vi "tensiletestpractice.vi"() -> ()   [LabVIEW 2014]
uses:
  <vilib>/Motion/FlexMotion/CustomControls/CustomControls.llb/Axis To Control.flx
  <vilib>/Motion/FlexMotion/FunctionsVIs/StartStopMotion.llb/Start Motion (8 axes).flx
  <vilib>/Motion/FlexMotion/FunctionsVIs/Trajectory.llb/Check Move Complete Status (8 axes).flx
  <vilib>/Motion/FlexMotion/FunctionsVIs/StartStopMotion.llb/Stop Motion (8 axes).flx
  Instance           1 22Saved   membrane_test3 .vi
  <vilib>/addons/_office/excel.llb/Excel Easy Table (num).vi
  <vilib>/Utility/NIReport.llb/NI_report.lvclass
  <vilib>/vision/NI_Vision_Development_Module.lvlib
  <vilib>/addons/_office/NI_ReportGenerationToolkit.lvlib
panel:
  out "?":string
  in  "Zero":dbl=-99.6 format="%#_13g"
  in  "Stretch Ratio Muliplier Per Cycle After":dbl=1.0 min=1.0
  in  "Number of cycles at 1x stretch ratio":dbl
  out "Waveform Chart":dynamicdata(graph)
  out "Finished at (s)":dbl format="%0.3f"
  in  "?":bool
  in  "Input File Path":path=path "C:/Users/aldasou3.ME204/Desktop/information.txt"
  out "Stretch length (mm)":dbl
  out "Estimated time from\nStart to finish (s)":dbl
  out "Elapsed Time (s)":dbl format="%0.3f"
  in  "Number of cycles":dbl
  in  "Stretch ratio":dbl
  in  "Motor speed\n(mm/s)":dbl
  in  "Undeformed\nLength (mm)\n(post to post)":dbl
  out "Voltage(V)":dbl=0.3869919147841388
  out "Particle Coordinates":dbl[][](array[numeric])
  out "Force (grams)":dbl=0.3869919147841388
  out "Selected Region of Interest":T1(plugin-control)
  out "Binary/ Segmented Image":T1(plugin-control)
  # "Michigan State University\nDepartment of Mechanical Engineering\nSoft Tissues Research Laboratory"
  # "Tensile Test and Particle Tracking VI"
  # "Image  Acquisition and Processing"
  # "Motion Control"
  # "Inputs"
  # "Selected Region of Interest"
  # "Experimental Data"
  # "Binary/Segmented Image"
  # "Distance between dots(mm)"
  # "1"
  # "2"
  # "3"
  # "4"
  # "Button must be white to run"
  # "5"
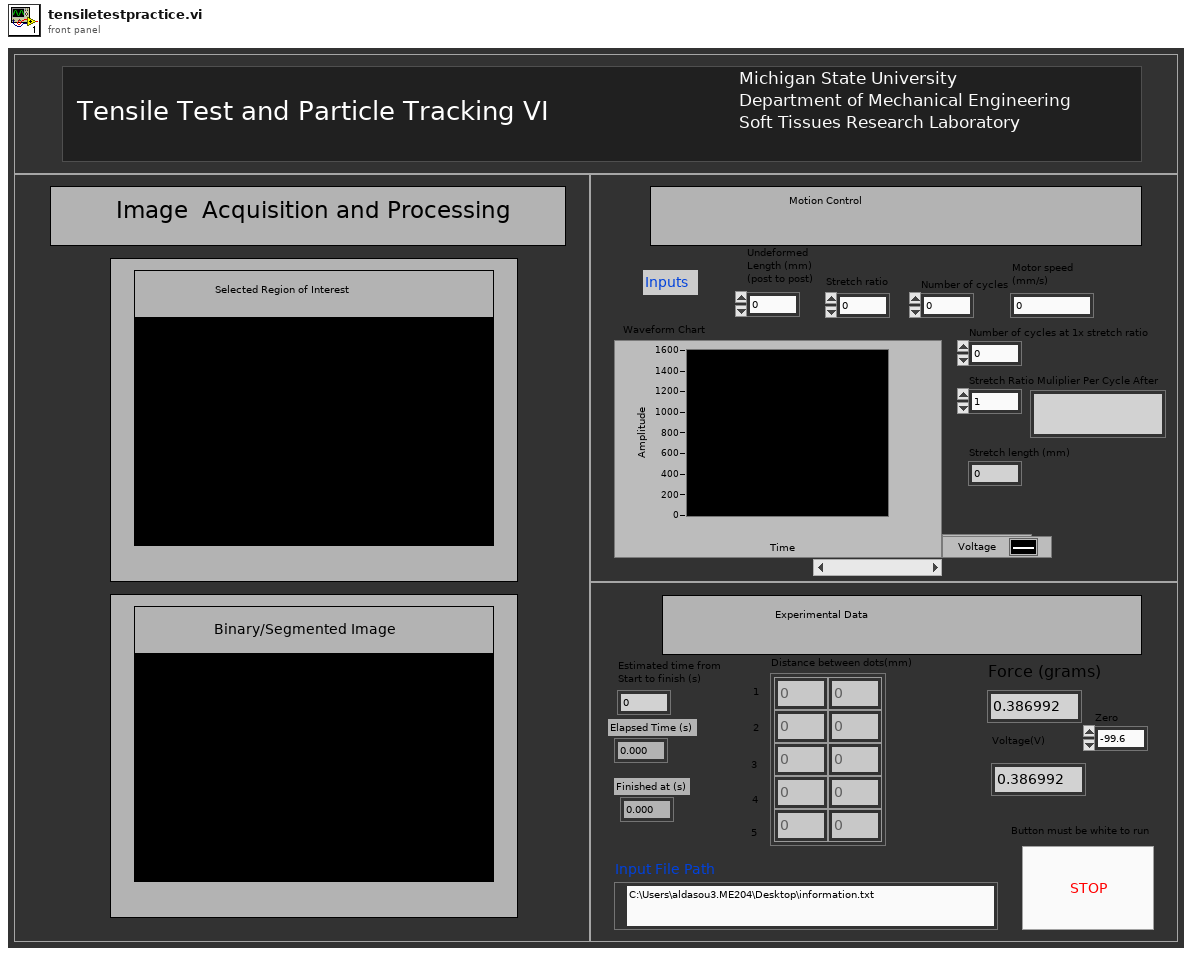
[diagram p1: front panel]
types:
  T1 = typedef "IMAQ Image.ctl" = refnum<image>
  T2 = typedef "Board Id" = u8
  T3 = enum16{"Absolute Position", "Relative Position", "Velocity", "Relative to Cap Pos", "Modulus Position", "Absolute Contouring", "Relative Contouring"}
  T4 = enum16{"Standard Report", "HTML", "Word", "Excel"}
  T5 = typedef "ROI Descriptor" = cluster{"Global Rectangle":i32[], "Contours":cluster{"ID":enum32{"External", "Internal"}, "Type":u32, "Coordinates":i32[]}[]}
  T6 = typedef "Axis To Control.flx" = u16
  T7 = typedef "Bd Id Out" = u8
  T8 = typedef "Resource Out (Enum).flx" = u16
  T9 = typedef "LVDateTimeRec.ctl" = cluster{"fractional second":dbl, "second":i32, "minute":i32, "hour":i32, "day of month":i32, "month":i32, "year":i32, "day of week":i32, "day of year":i32, "DST":i32}
  T10 = cluster{"month":i32, "day of month":i32, "year":i32, "hour":i32, "minute":i32, "second":i32}
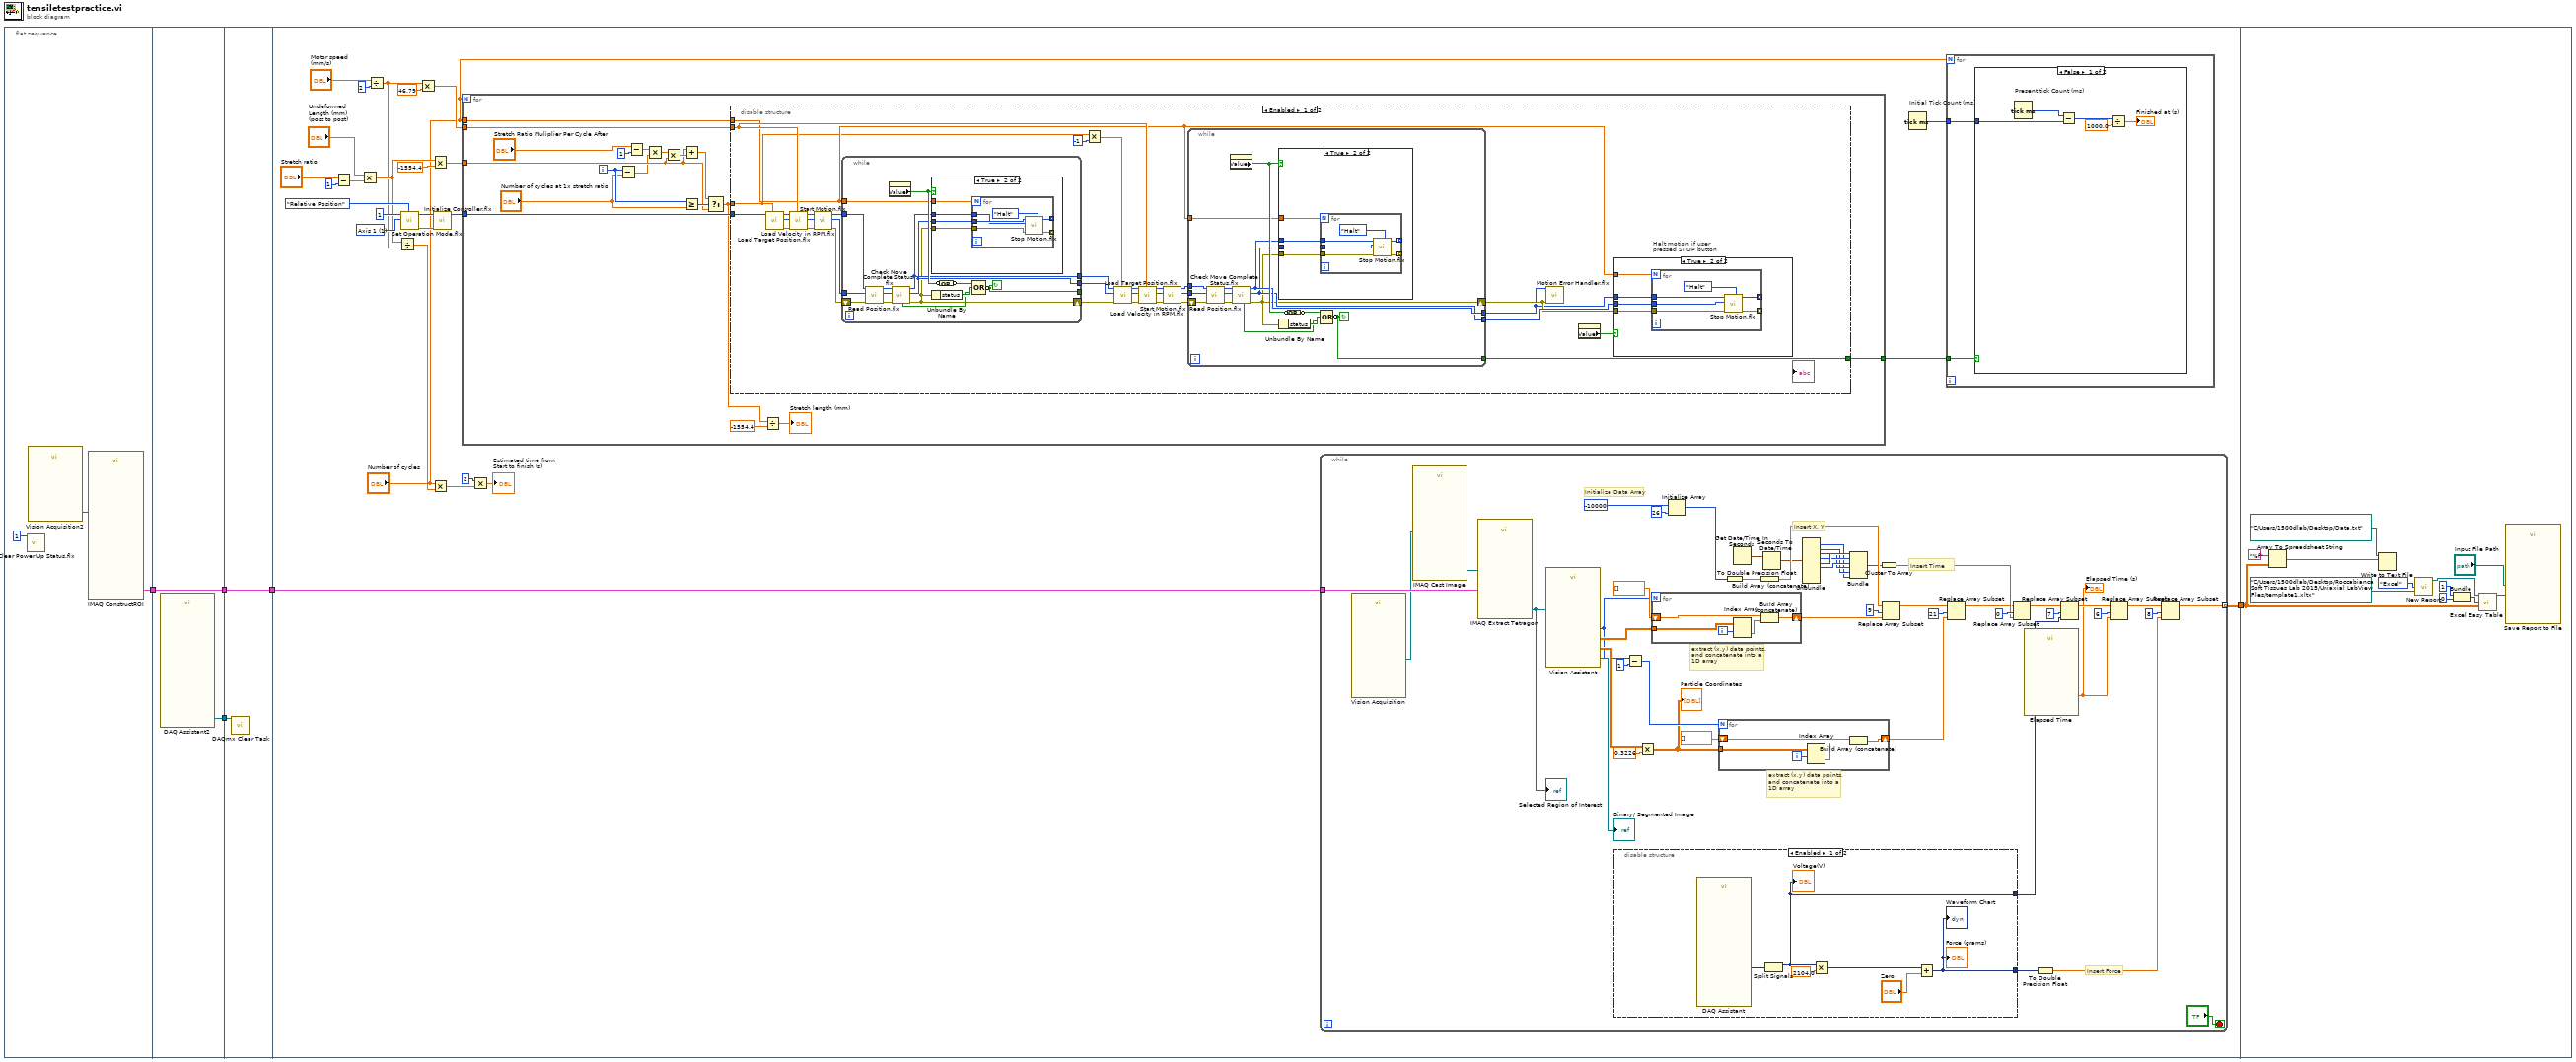
[diagram p0: block diagram]
diagram:
  n1 = flat-sequence {
    tunnel: [w7] -> w5
    tunnel: w5 -> [w10]
    tunnel: [w10] -> w4
    tunnel: [w9] -> w2
    tunnel: w4 -> [w12]
    tunnel: [w12] -> w3
    tunnel: w2 -> [w11]
    tunnel: w3 -> [w24]
    tunnel: [w21] -> w1
    tunnel: w1 -> [w223]
    frame #0 {
      n2 = call <vilib>:"Clear Power Up Status.flx"("Board ID"=1) -> ()  [unwired: 6 in, 2 out]
      n3 = call "Vision Acquisition2"() -> ("Image Out"=w8:T1)  [unwired: 26 in, 1 out]
      n4 = call "IMAQ ConstructROI"("Image"=w8) -> ("ROI Descriptor Out"=w7:T5)  [unwired: 7 in, 3 out]
    }
    frame #1 {
      n5 = call "DAQ Assistant2"() -> ("task out"=w9:refnum<k21>)  [unwired: 16 in, 3 out]
    }
    frame #2 {
      n6 = call <vilib>:"DAQmx Clear Task.vi"("task in"=w11) -> ()  [unwired: 14 in, 1 out]
    }
    frame #3 {
      w34 = T6 1 items=["Axis 1"=1, "Axis 2"=2, "Axis 3"=3, "Axis 4"=4, "Axis 5"=5, "Axis 6"=6, "Axis 7"=7, "Axis 8"=8] ("Axis")
      n7 = Subtract(x="Stretch ratio", y=1) -> (x-y=w14:dbl)
      n8 = Multiply(x="Undeformed\nLength (mm)\n(post to post)", y=w14) -> (x*y=w28:dbl)
      n9 = Divide(x="Motor speed\n(mm/s)", y=2) -> (x/y=w20:dbl)
      n10 = Divide(x=w28, y=w20) -> (x/y=w27:dbl)
      n11 = call <vilib>:"Set Operation Mode.flx"("Position Mode (Absolute)"=T3."Relative Position", "Axis or Vector Space"=w34, "Board ID"=T2 1) -> ("error out"=w35:errorcluster, "Bd ID Out"=w36:T7)  [unwired: 3 in, 1 out]
      n12 = Multiply(x=w20, y=46.79) -> (x*y=w31:dbl)
      n13 = Multiply(x=w28, y=-1554.4) -> (x*y=w26:dbl)
      n14 = Multiply(x="Number of cycles", y=w27) -> (x*y=w18:dbl)
      n15 = call <vilib>:"Initialize Controller.flx"("error in (no error)"=w35, "Board ID"=w36) -> ("Bd ID Out"=w29:T7)  [unwired: 6 in, 1 out]
      n16 = for {
        N: "Number of cycles" -> [_]
        tunnel: w31 -> [w64]
        tunnel: w26 -> [w54]
        tunnel: w29 -> [w63]
        tunnel: [w62] -> w25
        tunnel: "Number of cycles" -> [w61]
        i -> [w49]
        n17 = Subtract(x=w49, y="Number of cycles at 1x stretch ratio") -> (x-y=w47:dbl)
        n18 = Subtract(x="Stretch Ratio Muliplier Per Cycle After", y=1) -> (x-y=w50:dbl)
        n19 = Multiply(x=w50, y=w47) -> (x*y=w56:dbl)
        n20 = Multiply(x=w56, y=w54) -> (x*y=w55:dbl)
        n21 = Add(x=w54, y=w55) -> (x+y=w53:dbl)
        n22 = Greater Or Equal?(x=w49, y="Number of cycles at 1x stretch ratio") -> (x >= y?=w57:bool)
        n23 = Select(t=w53, s=w57, f=w54) -> (s? t:f=w60:dbl)
        n24 = disable-structure shown="Enabled" {
          disable-tunnel: w64 -> [w74 _]
          disable-tunnel: w60 -> [w65 _]
          disable-tunnel: w63 -> [w75 _]
          disable-tunnel: [w70 _] -> w62
          disable-tunnel: w61 -> [w69 _]
          frame Enabled {
            # "Halt motion if user\npressed STOP button"
            n25 = call <vilib>:"Load Target Position.flx"("Target Position (0)"=w65, "Board ID"=w75) -> ("error out"=w94:errorcluster, "Resource Output"=w95:T8, "Bd ID Out"=w96:T7)  [unwired: 5 in]
            n26 = call <vilib>:"Load Velocity in RPM.flx"("Velocity (500)"=w74, "error in (no error)"=w94, "Axis or Vector Space"=w95, "Board ID"=w96) -> ("error out"=w89:errorcluster, "Resource Output"=w73:T8, "Bd ID Out"=w90:T7)  [unwired: 3 in]
            n27 = call-poly <vilib>:"Start Motion.flx"("error in (no error)"=w89, "Axis or Vector Space"=w73, "Board ID"=w90) -> ("error out"=w93:errorcluster, "Resource Output"=w92:T8, "Bd ID Out"=w91:T7)  [unwired: 3 in]
            n28 = while {
              tunnel: [w133] -> w81
              shift-left: w93 -> [w139]
              shift-right: [w132] -> w80
              tunnel: [w134] -> w82
              tunnel: w92 -> [w145]
              tunnel: w91 -> [w140]
              tunnel: [w138] -> _
              tunnel: w69 -> [w135]
              stop <- w138 continue-if-true
              n29 = call <vilib>:"Read Position.flx"("error in (no error)"=w139, "Axis"=w145, "Board ID"=w140) -> ("error out"=w143:errorcluster, "Resource Output"=w144:T8, "Bd ID Out"=w146:T7)  [unwired: 3 in, 1 out]
              n30 = property class="Bool (strict)"() -> ("Value"=w136:bool)  [unwired: 2 in, 2 out]
              n31 = call-poly <vilib>:"Check Move Complete Status.flx"("error in (no error)"=w143, "Axis or Vector Space"=w144, "Board ID"=w146) -> ("error out"=w132:errorcluster, "Resource Output"=w133:T8, "Bd ID Out"=w134:T7, "Move Complete"=w141:bool)  [unwired: 3 in]
              n32 = case shown="True" w136 {
                tunnel: w134 -> [_ w150]
                tunnel: w132 -> [_ w149]
                tunnel: w133 -> [_ w148]
                tunnel: w135 -> [_ w147]
                frame False {
                }
                frame True {
                  n33 = for {
                    N: w147 -> [_]
                    tunnel: w150 -> [w155]
                    tunnel: w149 -> [w154]
                    tunnel: [w153] -> _ mode=indexing
                    tunnel: [w152] -> _ mode=indexing
                    tunnel: w148 -> [w151]
                    n34 = call-poly <vilib>:"Stop Motion.flx"("Stop Type (Decel)"=enum16{"Decelerate", "Halt", "Kill"}."Halt", "error in (no error)"=w154, "Axis or Vector Space"=w151, "Board ID"=w155) -> ("error out"=w153:errorcluster, "Bd ID Out"=w152:T7)  [unwired: 3 in, 1 out]
                  }
                }
              }
              n35 = Unbundle By Name(w132) -> ("status"=w142:bool)
              n36 = Compound Arithmetic op=OR(invert w136) -> (invert w137:bool)
              n37 = Compound Arithmetic op=OR(w137, w142, w141) -> (invert w138:bool)
            }
            n38 = Multiply(x=w65, y=-1) -> (x*y=w66:dbl)
            n39 = call <vilib>:"Load Target Position.flx"("Target Position (0)"=w66, "error in (no error)"=w80, "Axis"=w81, "Board ID"=w82) -> ("error out"=w86:errorcluster, "Resource Output"=w87:T8, "Bd ID Out"=w88:T7)  [unwired: 3 in]
            n40 = call <vilib>:"Load Velocity in RPM.flx"("Velocity (500)"=w74, "error in (no error)"=w86, "Axis or Vector Space"=w87, "Board ID"=w88) -> ("error out"=w84:errorcluster, "Resource Output"=w83:T8, "Bd ID Out"=w85:T7)  [unwired: 3 in]
            n41 = call-poly <vilib>:"Start Motion.flx"("error in (no error)"=w84, "Axis or Vector Space"=w83, "Board ID"=w85) -> ("error out"=w79:errorcluster, "Resource Output"=w78:T8, "Bd ID Out"=w77:T7)  [unwired: 3 in]
            n42 = while {
              tunnel: [w108] -> w76
              shift-left: w79 -> [w114]
              shift-right: [w107] -> w72
              tunnel: [w109] -> w71
              tunnel: w78 -> [w120]
              tunnel: w77 -> [w115]
              tunnel: [w113] -> w70
              tunnel: w69 -> [w110]
              stop <- w113 continue-if-true
              n43 = call <vilib>:"Read Position.flx"("error in (no error)"=w114, "Axis"=w120, "Board ID"=w115) -> ("error out"=w118:errorcluster, "Resource Output"=w119:T8, "Bd ID Out"=w121:T7)  [unwired: 3 in, 1 out]
              n44 = property class="Bool (strict)"() -> ("Value"=w111:bool)  [unwired: 2 in, 2 out]
              n45 = call-poly <vilib>:"Check Move Complete Status.flx"("error in (no error)"=w118, "Axis or Vector Space"=w119, "Board ID"=w121) -> ("error out"=w107:errorcluster, "Resource Output"=w108:T8, "Bd ID Out"=w109:T7, "Move Complete"=w116:bool)  [unwired: 3 in]
              n46 = case shown="True" w111 {
                tunnel: w109 -> [_ w125]
                tunnel: w107 -> [_ w124]
                tunnel: w108 -> [_ w123]
                tunnel: w110 -> [_ w122]
                frame False {
                }
                frame True {
                  n47 = for {
                    N: w122 -> [_]
                    tunnel: w125 -> [w130]
                    tunnel: w124 -> [w129]
                    tunnel: [w128] -> _ mode=indexing
                    tunnel: [w127] -> _ mode=indexing
                    tunnel: w123 -> [w126]
                    n48 = call-poly <vilib>:"Stop Motion.flx"("Stop Type (Decel)"=enum16{"Decelerate", "Halt", "Kill"}."Halt", "error in (no error)"=w129, "Axis or Vector Space"=w126, "Board ID"=w130) -> ("error out"=w128:errorcluster, "Bd ID Out"=w127:T7)  [unwired: 3 in, 1 out]
                  }
                }
              }
              n49 = Unbundle By Name(w107) -> ("status"=w117:bool)
              n50 = Compound Arithmetic op=OR(invert w111) -> (invert w112:bool)
              n51 = Compound Arithmetic op=OR(w112, w117, w116) -> (invert w113:bool)
            }
            n52 = call <vilib>:"Motion Error Handler.flx"("Board ID"=w71, "error in (no error)"=w72) -> ()  [unwired: 9 in, 5 out]
            n53 = property class="Bool (strict)"() -> ("Value"=w68:bool)  [unwired: 2 in, 2 out]
            n54 = case shown="True" w68 {
              tunnel: w71 -> [_ w100]
              tunnel: w72 -> [_ w99]
              tunnel: w76 -> [_ w98]
              tunnel: w69 -> [_ w97]
              frame False {
              }
              frame True {
                n55 = for {
                  N: w97 -> [_]
                  tunnel: w100 -> [w105]
                  tunnel: w99 -> [w104]
                  tunnel: [w103] -> _ mode=indexing
                  tunnel: [w102] -> _ mode=indexing
                  tunnel: w98 -> [w101]
                  n56 = call-poly <vilib>:"Stop Motion.flx"("Stop Type (Decel)"=enum16{"Decelerate", "Halt", "Kill"}."Halt", "error in (no error)"=w104, "Axis or Vector Space"=w101, "Board ID"=w105) -> ("error out"=w103:errorcluster, "Bd ID Out"=w102:T7)  [unwired: 3 in, 1 out]
                }
              }
            }
          }
          frame Disabled {
          }
        }
        n57 = Divide(x=w60, y=-1554.4) -> (x/y=→"Stretch length (mm)":dbl)
      }
      n58 = Multiply(x=2, y=w18) -> (x*y=→"Estimated time from\nStart to finish (s)":dbl)
      n59 = while {
        tunnel: w24 -> [w204]
        tunnel: [w162] -> w21 mode=indexing
        stop <- "?" stop-if-true
        # "extract (x,y) data points,\nand concatenate into a \n1D array"
        # "extract (x,y) data points,\nand concatenate into a \n1D array"
        # "Insert Force"
        # "Insert X, Y"
        # "Insert Time"
        # "Initialize Data Array"
        n60 = call "Vision Acquisition"() -> ("Image Out"=w200:T1)  [unwired: 24 in, 3 out]
        n61 = call "IMAQ Cast Image"("Image Src"=w200) -> ("Image Dst Out"=w201:T1)  [unwired: 9 in, 1 out]
        n62 = call-poly "IMAQ Extract Tetragon"("ROI Descriptor"=w204, "Image Src"=w201) -> ("Image Dst Out"=w202:T1)  [unwired: 8 in, 1 out]
        "Selected Region of Interest" <- w202
        n63 = call "Vision Assistant"("Image In"=w202) -> ("Image Out"=→"Binary/ Segmented Image":T1, "Particle Measurements (Pixels) (Particle Analysis 2)"=w161:dbl[][], "Number of Particles (Particle Analysis 2)"=w158:i32, "Caliper Results (Caliper 1)"=w168:sgl[][])  [unwired: 22 in, 1 out]
        n64 = disable-structure shown="Enabled" {
          disable-tunnel: [w215 _] -> w190
          disable-tunnel: [w216 _] -> w175
          frame Enabled {
            n65 = call "DAQ Assistant"() -> ("data"=w217:dynamicdata)  [unwired: 16 in, 3 out]
            n66 = Split Signals(w217) -> (w216:dynamicdata)  [unwired: 2 in, 1 out]
            "Voltage(V)" <- w216
            n67 = Multiply(x=w216, y=2104.0) -> (x*y=w220:dynamicdata)
            n68 = Add(x=w220, y="Zero") -> (x+y=w215:dynamicdata)
            "Force (grams)" <- w215
            "Waveform Chart" <- w215
          }
          frame Disabled {
          }
        }
        n69 = Subtract(x=w158, y=1) -> (x-y=w169:i32)
        n70 = Multiply(x=w168, y=0.3226) -> (x*y=w163:dbl[][])
        "Particle Coordinates" <- w163
        n71 = for {
          N: w158 -> [_]
          shift-right: [w212] -> w167
          shift-left: dbl[] [] -> [w213]
          tunnel: w161 -> [w210]
          i -> [w214]
          n72 = Index Array(array=w210, index (row)=w214) -> (element=w211:dbl[])  [unwired: 1 in]
          n73 = Build Array (concatenate)(w213, w211) -> (w212:dbl[])
        }
        n74 = Initialize Array(-10000, 26) -> (w196:i32[])
        n75 = for {
          N: w169 -> [_]
          shift-right: [w207] -> w166
          shift-left: dbl[] [] -> [w208]
          tunnel: w163 -> [w205]
          i -> [w209]
          n76 = Index Array(array=w205, index (row)=w209) -> (element=w206:dbl[])  [unwired: 1 in]
          n77 = Build Array (concatenate)(w208, w206) -> (w207:dbl[])
        }
        n78 = To Double Precision Float(number=w196) -> (double precision float=w197:dbl[])
        n79 = Get Date/Time In Seconds() -> (seconds since 1Jan1904=w187:timestamp)
        n80 = Build Array (concatenate)(w197) -> (w192:dbl[])
        n81 = Seconds To Date/Time(time stamp (now)=w187) -> (date time rec=w186:T9)  [unwired: 1 in]
        n82 = Unbundle(w186) -> ("second"=w177:i32, "minute"=w178:i32, "hour"=w179:i32, "day of month"=w181:i32, "month"=w182:i32, "year"=w180:i32)  [unwired: 4 out]
        n83 = Bundle("month"=w182, "day of month"=w181, "year"=w180, "hour"=w179, "minute"=w178, "second"=w177) -> (w184:T10)  [unwired: 1 in]
        n84 = Cluster To Array(cluster=w184) -> (array=w183:i32[])
        n85 = Replace Array Subset(array=w192, new element=w167, index=9) -> (w165:dbl[])
        n86 = Replace Array Subset(array=w165, new element=w166, index=21) -> (w164:dbl[])
        n87 = Replace Array Subset(array=w164, new element=w183, index=0) -> (w174:dbl[])
        n88 = call "Elapsed Time"() -> ("Elapsed Time (s)"=w157:dbl)  [unwired: 12 in, 7 out]
        "Elapsed Time (s)" <- w157
        n89 = To Double Precision Float(number=w190) -> (double precision float=w189:dbl)
        n90 = Replace Array Subset(array=w174, new element=w175, index=7) -> (w173:dbl[])
        n91 = Replace Array Subset(array=w173, new element=w157, index=6) -> (w188:dbl[])
        n92 = Replace Array Subset(array=w188, new element=w189, index=8) -> (w162:dbl[])
      }
      n93 = Tick Count (ms) "Initial Tick Count (ms)"() -> (millisecond timer value=w23:u32)
      n94 = for {
        N: "Number of cycles" -> [_]
        tunnel: w23 -> [w41]
        tunnel: w25 -> [w40]
        n95 = case shown="False" w40 {
          tunnel: w41 -> [w42 _]
          frame False {
            n96 = Tick Count (ms) "Present tick Count (ms)"() -> (millisecond timer value=w45:u32)
            n97 = Subtract(x=w45, y=w42) -> (x-y=w46:u32)
            n98 = Divide(x=w46, y=1000.0) -> (x/y=→"Finished at (s)":dbl)
          }
          frame True {
          }
        }
      }
    }
    frame #4 {
      n99 = Array To Spreadsheet String(array=w223, 3:"%f" ("format string")) -> (spreadsheet string=w227:string)  [unwired: 1 in]
      n100 = Write to Text File(file (use dialog)=path "C:/Users/1500dlab/Desktop/Data.txt" ("file path"), text=w227) -> ()  [unwired: 2 in, 3 out]
      n101 = call <vilib>:"New Report.vi"("report type"=T4."Excel", "template (empty)"=path "C:/Users/1500dlab/Desktop/Roccabianca Soft Tissues Lab 2015/Uniaxial LabView Files/template1.xltx" ("file path")) -> ("report out"=w222:refnum<class "NI_report.lvclass">)  [unwired: 12 in, 1 out]
      n102 = Bundle(1, 0) -> (w228:cluster{i32, i32})  [unwired: 1 in]
      n103 = call-poly <vilib>:"Excel Easy Table.vi"("report in"=w222, "start (0, 0)"=w228, "text data"=w223) -> ("report out"=w231:refnum<class "NI_report.lvclass">)  [unwired: 8 in, 4 out]
      n104 = call-dynamic "Save Report to File.vi"("report in"=w231, "report file path"="Input File Path") -> ()  [unwired: 12 in, 2 out]
    }
  }
